vi "Configure MCCW Crest Factor Mode.vi"(8 "error in (no error)":errorcluster, 9 "Crest factor target":dbl, 10 "Crest factor mode":enum16{"Off", "Chirp", "Slow"}(ring), 11 "VSG-SMBV in":refnum<class "VSG-SMBV.lvclass">) -> (0 "error out":errorcluster, 3 "VSG-SMBV out":refnum<class "VSG-SMBV.lvclass">)   [LabVIEW 2020, in "VSG-SMBV.lvclass"]
doc: "Configure the crest factor optimazation mode"
uses:
  VSG-SMBV.lvclass
  C:/Sandbox/RF Bench/Source Code/WiSpry Test Framework/Instruments/Instrument.lvclass
  Instrument.lvclass/Instrument.ctl
  Instrument.lvclass
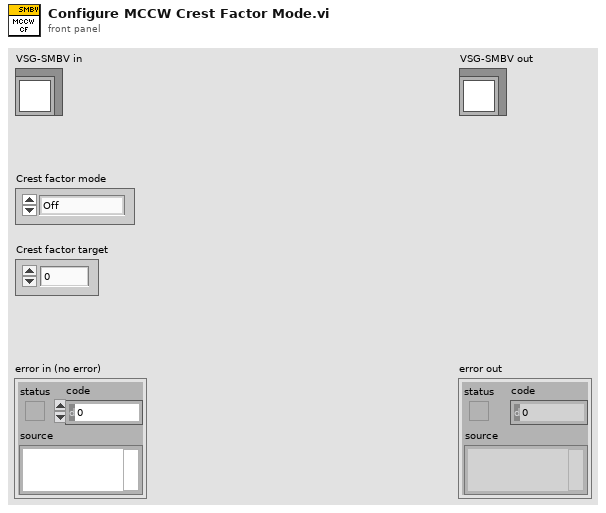
[diagram p1: front panel]
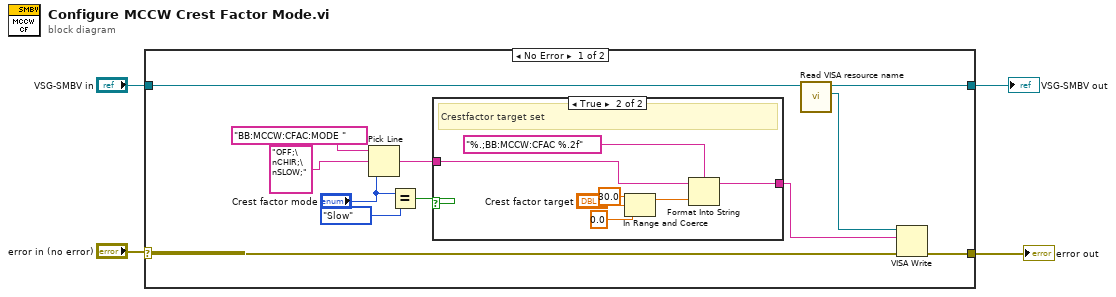
[diagram p0: block diagram]
diagram:
  n1 = case shown="No Error" "error in (no error)" {
    selector: "error in (no error)" -> [w9 w26]
    tunnel: "VSG-SMBV in" -> [w10 w25]
    tunnel: [w6 w26] -> w2
    tunnel: [w5 w25] -> w1
    frame No Error {
      n2 = Pick Line(string ("")="BB:MCCW:CFAC:MODE ", multi-line string="OFF;\nCHIR;\nSLOW;", line index="Crest factor mode") -> (output string=w11:string)
      n3 = Equal?(x="Crest factor mode", y=enum16{"Off", "Chirp", "Slow"}."Slow") -> (x = y?=w12:bool)
      n4 = case shown="True" w12 {
        tunnel: w11 -> [w17 w24]
        tunnel: [w17 w18] -> w7
        frame False {
          # "Crest factor ignored"
        }
        frame True {
          # "Crestfactor target set"
          n5 = In Range and Coerce(upper limit=30.0, x="Crest factor target", lower limit=0.0) -> (coerced(x)=w19:dbl)  [unwired: 1 out]
          n6 = Format Into String(format string="%.;BB:MCCW:CFAC %.2f", initial string=w24, w19) -> (resulting string=w18:string)  [unwired: 1 in, 1 out]
        }
      }
      n7 = call "Read VISA resource name.vi"("Instrument in"=w10) -> ("VISA resource name"=w8:refnum<visa-resource-name>, "Instrument out"=w5:refnum<class "VSG-SMBV.lvclass">)  [unwired: 9 in]
      n8 = VISA Write(VISA resource name=w8, write buffer=w7, error in (no error)=w9) -> (error out=w6:errorcluster)  [unwired: 2 out]
    }
    frame Error {
    }
  }
  "error out" <- w2
  "VSG-SMBV out" <- w1
